vi "test_232-GNSS_gmap.vi"() -> ()   [LabVIEW 2019]
uses:
  Ctrl/gnss_config.ctl
  C:/Users/wego/Documents/GitHub/Ycar/LabVIEW/Gmap/dll/GMap.NET.WindowsForms.dll
  Gmap/dll/GMap.NET.WindowsForms.dll
  Ctrl/ublox-ui_main.ctl
  Ctrl/cmd_common.ctl
  Gmap/gmap_fgv-cmd.ctl
  Gmap/marker_info.ctl
panel:
  in  "탭":enum32{"Main", "설정"}(tab)
  in  "GMapControl":refnum<k24>(container)
  out "TM graph":T1(graph)
  in  "stop":bool
  in  "zoom":dbl(slide) scale=3.0..20.0
  in  "gmap center":bool
  in  "PinDropMrkr":T2(ring)=enum."red_dot" caption="Pin Drop Marker"
  out "error out":errorcluster
  out "n":i32
  out "read_buffer raw":string
  out "Arr-size":i32
  out "xcenter_TM":dbl
  out "ycenter_TM":dbl
  out "R_TM":dbl
  out "ublox info":T3 {"HDOP" scale=0.0..10.0; "PDOP" scale=0.0..10.0; "2D Acc.m" scale=0.0..10.0; "Latitude" format="%.9f"; "Longitude" format="%.9f"; "3D Acc.m" scale=0.0..10.0}
  in  "Map Lon":dbl format="%.11f"
  in  "Map Lat":dbl format="%.11f"
  out "read_buffer":string
  in  "GNSS cfg":T4={"Port"="COM10", "heading select"="", "PwrPak7_mode select"=[], "rate"=115200}
  out "buffer n":u32(graph)
  in  "Lon Dbclk":dbl format="%.11f"
  in  "Lat Dbclk":dbl format="%.11f"
  out "val":bool
  in  "sel":T5(ring)=enum."GxGGA"
  in  "index latlong":T6={"lat_index"=1, "lon_index"=3, "heading index"=0}
  in  "log":bool
  out "TM array":cluster{"Y(E)":dbl, "X(N)":dbl}[](array[cluster])
  in  "arr limit":i32=200
  # "GNSS/GPS Test Program"
  # "GPS/GNSS 테스트 프로그램"
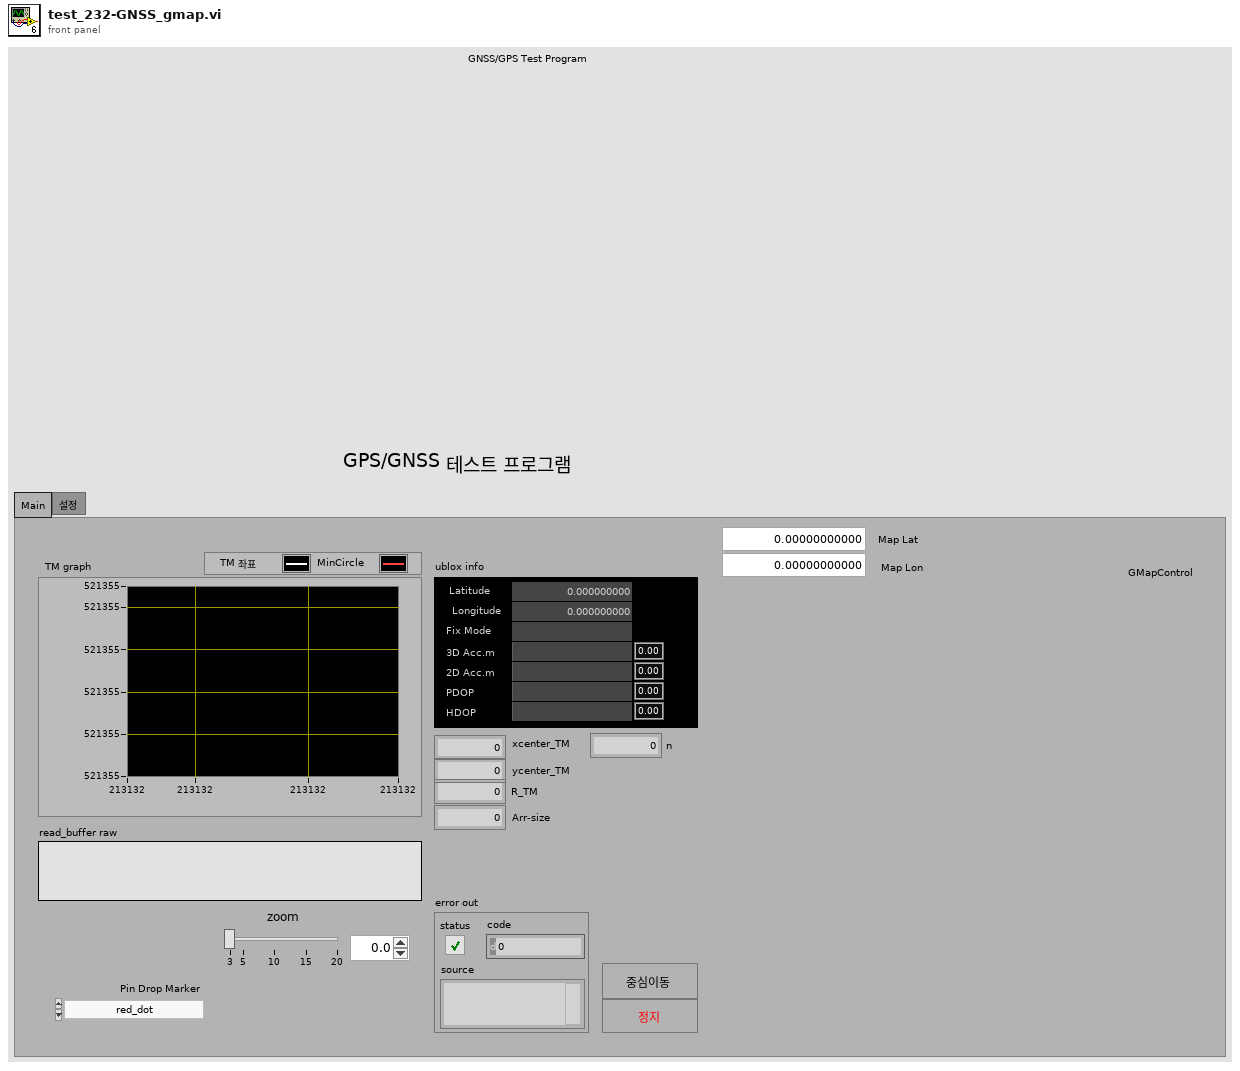
[diagram p1: front panel]
types:
  T1 = cluster{"TM array":cluster{"Y(E)":dbl, "X(N)":dbl}[]}[]
  T2 = enum16{"none", "arrow", "blue", "blue_small", "blue_dot", "blue_pushpin", "brown_small", "gray_small", "green", "green_small", "green_dot", "green_pushpin", "green_big_go", "yellow", "yellow_small", "yellow_dot", "yellow_big_pause", "yellow_pushpin", "lightblue", "lightblue_dot", "lightblue_pushpin", "orange", "orange_small", "orange_dot", "pink", "pink_dot", "pink_pushpin", "purple", "purple_small", "purple_dot", "purple_pushpin", "red", "red_small", "red_dot", "red_pushpin", "red_big_stop", "black_small", "white_small"}
  T3 = typedef "ublox-ui_main.ctl" = cluster{"Latitude":dbl, "Longitude":dbl, "Fix Mode":string, "3D Acc.m":dbl, "2D Acc.m":dbl, "PDOP":dbl, "HDOP":dbl}
  T4 = typedef "gnss_config.ctl" = cluster{"Port":refnum<visa-resource-name>, "heading select":string, "PwrPak7_mode select":string[], "rate":u32}
  T5 = enum16{"GxDTM", "GxGBS", "GxGGA", "GxGLL", "GxGNS", "GxGRS", "GxGSA", "GxGST", "GxGSV", "GxRLM", "GxRMC", "GxTHS", "GxTXT", "GxVLW", "GxVTG", "GxZDA"}
  T6 = cluster{"lat_index":i32, "lon_index":i32, "heading index":i32}
  T7 = typedef "cmd_common.ctl" = enum16{"read", "write"}
  T8 = cluster{"Map Lat":refnum<vi>, "Map Lon":refnum<vi>, "Lat Dbclk":refnum<vi>, "Lon Dbclk":refnum<vi>, "zoom":refnum<vi>, "PinDropMrkr":refnum<vi>}
  T9 = typedef "gmap_fgv-cmd.ctl" = enum16{"marker type change", "save_image", "coll of points", "zoom n center markers", "add overlay reference", "read", "zoom", "set position by keyword", "set map provider", "map provider update", "create", "add marker", "clear marker", "close"}
  T10 = typedef "marker_info.ctl" = cluster{"arrLatLngActv":dbl[], "type":i32}
  T11 = cluster{"TM array":cluster{"Y(E)":dbl, "X(N)":dbl}[]}
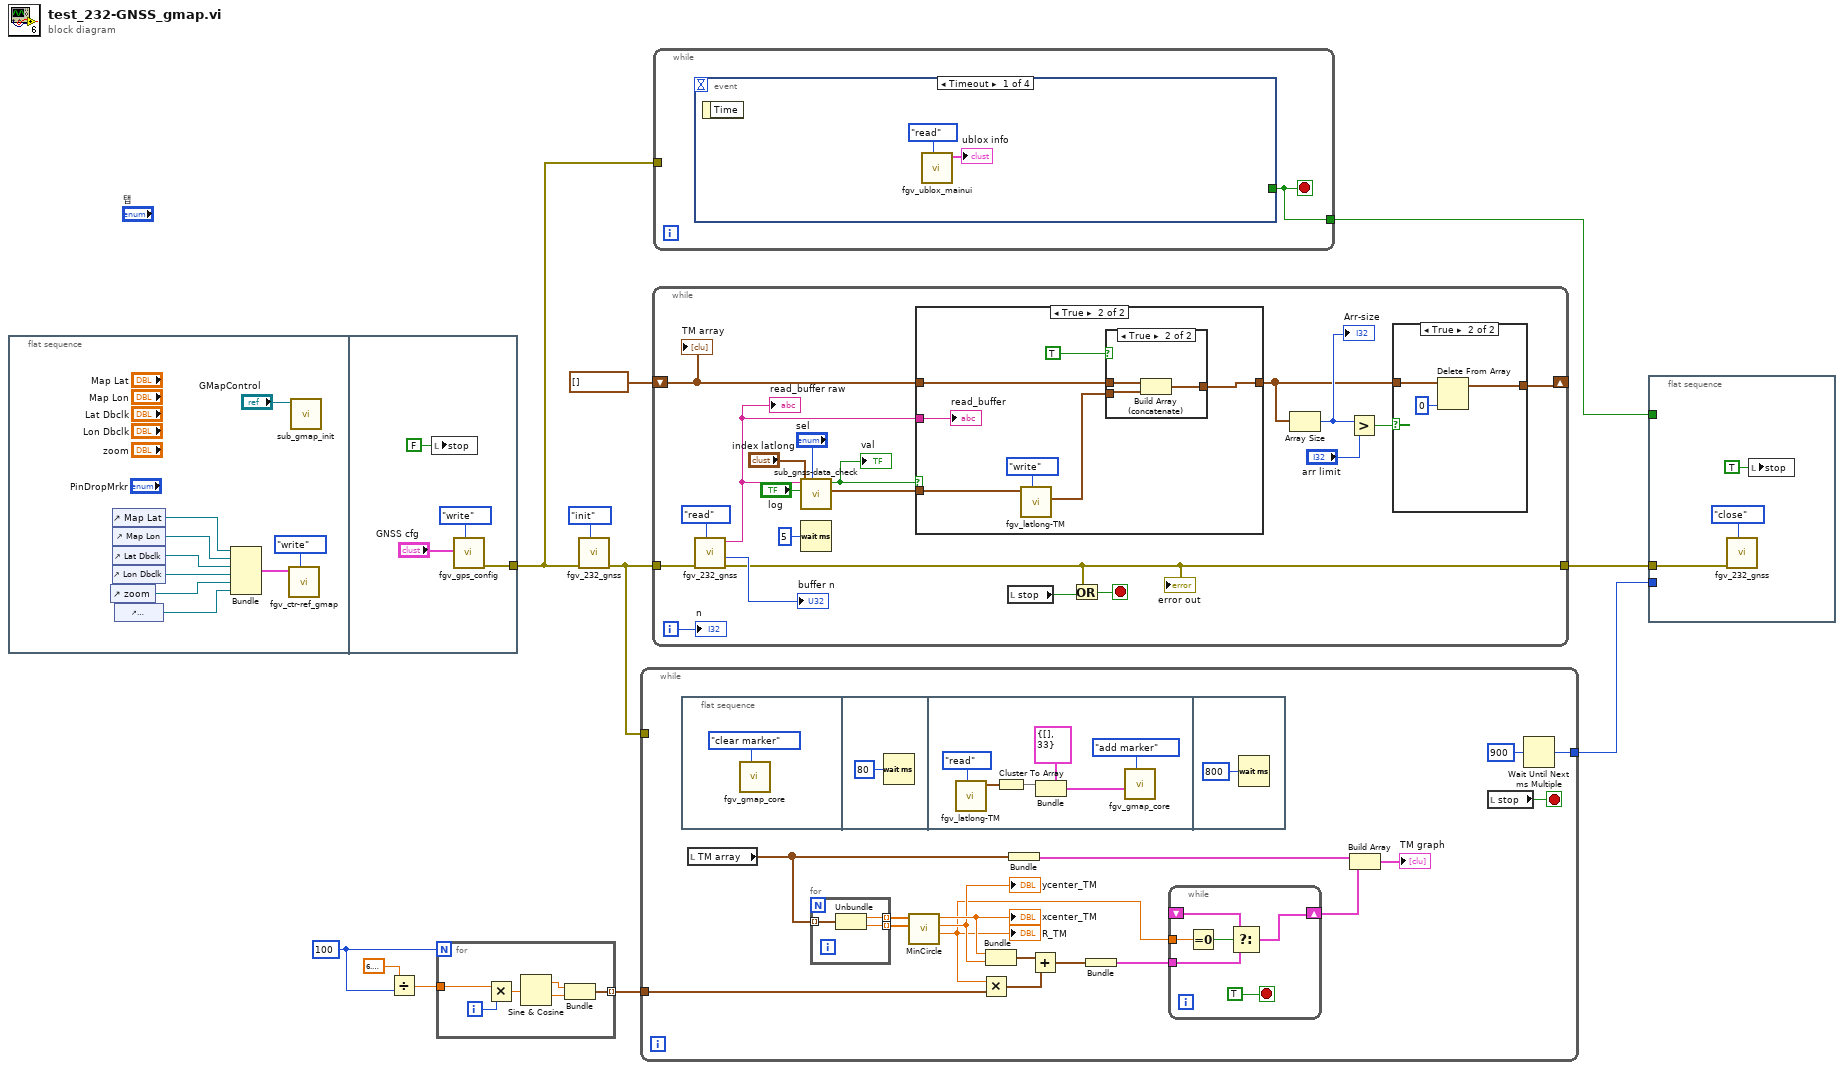
[diagram p0: block diagram]
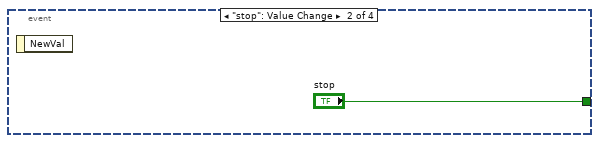
[diagram p2: hidden frame]
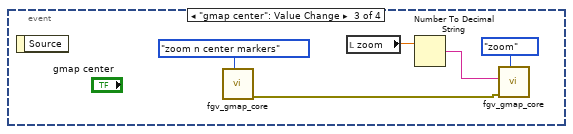
[diagram p3: hidden frame]
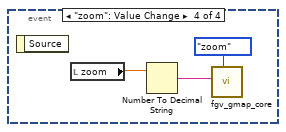
[diagram p4: hidden frame]
diagram:
  w3 = 100
  n1 = flat-sequence {
    tunnel: [w23] -> w7
    frame #0 {
      n2 = control-ref of="zoom"() -> (w13:refnum<vi>)
      n3 = control-ref of="Map Lat"() -> (w17:refnum<vi>)
      n4 = control-ref of="Map Lon"() -> (w16:refnum<vi>)
      n5 = control-ref of="Lat Dbclk"() -> (w15:refnum<vi>)
      n6 = control-ref of="Lon Dbclk"() -> (w14:refnum<vi>)
      n7 = control-ref of="PinDropMrkr"() -> (w12:refnum<vi>)
      n8 = Bundle("Map Lat"=w17, "Map Lon"=w16, "Lat Dbclk"=w15, "Lon Dbclk"=w14, "zoom"=w13, "PinDropMrkr"=w12) -> (w19:T8)  [unwired: 1 in]
      n9 = call "fgv_ctr-ref_gmap.vi"("cmd"=cmd_common."write", "ref in"=w19) -> ()  [unwired: 9 in, 1 out]
      n10 = call "sub_gmap_init.vi"("GMapControl"="GMapControl") -> ()  [unwired: 10 in, 1 out]
    }
    frame #1 {
      n11 = local write "stop"(FALSE ("정지")) -> ()
      n12 = call "fgv_gps_config.vi"("cmd"=enum16{"read", "write"}."write", "GNSS cfg"="GNSS cfg") -> ("error out"=w23:errorcluster)  [unwired: 8 in, 1 out]
    }
  }
  n13 = Divide(x=6.283185307179586, y=w3) -> (x/y=w4:dbl)
  n14 = for {
    N: w3 -> [_]
    tunnel: w4 -> [w29]
    tunnel: [w25] -> w1 mode=indexing
    i -> [w30]
    n15 = Multiply(x=w29, y=w30) -> (x*y=w28:dbl)
    n16 = Sine & Cosine(0:w28) -> (1:w27:dbl, 2:w26:dbl)
    n17 = Bundle(w27, w26) -> (w25:cluster{dbl, dbl})  [unwired: 1 in]
  }
  n18 = call "fgv_232_gnss.vi"("cmd"=enum16{"init", "read", "write", "close"}."init", "error in"=w7) -> ("error out"=w8:errorcluster)  [unwired: 7 in, 2 out]
  n19 = while {
    tunnel: w8 -> [_]
    tunnel: [w45] -> w6
    tunnel: w1 -> [w40]
    stop <- w47 stop-if-true
    n20 = flat-sequence {
      frame #0 {
        n21 = call "fgv_gmap_core.vi"("cmd"=gmap_fgv-cmd."clear marker") -> ()  [unwired: 7 in, 4 out]
      }
      frame #1 {
        n22 = Wait (ms)(milliseconds to wait=u32 80 ("대기 시간 (ms)")) -> ()  [unwired: 1 out]
      }
      frame #2 {
        n23 = call "fgv_latlong-TM.vi"("cmd"=enum16{"write", "read"}."read") -> ("latlong out"=w59:cluster{"lat":dbl, "long":dbl})  [unwired: 9 in, 1 out]
        n24 = Cluster To Array(cluster=w59) -> (array=w63:dbl[])
        n25 = Bundle(cluster=T10 {"arrLatLngActv"=[], "type"=33} ("marker_info"), "arrLatLngActv"=w63) -> (w61:T10)  [unwired: 1 in]
        n26 = call "fgv_gmap_core.vi"("cmd"=gmap_fgv-cmd."add marker", "marker_info"=w61) -> ()  [unwired: 6 in, 4 out]
      }
      frame #3 {
        n27 = Wait (ms)(milliseconds to wait=u32 800 ("대기 시간 (ms)")) -> ()  [unwired: 1 out]
      }
    }
    n28 = local read "TM array"() -> (w36:cluster{"Y(E)":dbl, "X(N)":dbl}[])
    n29 = for {
      tunnel: [w56] -> w44 mode=indexing
      tunnel: [w55] -> w43 mode=indexing
      tunnel: w36 -> [w54] mode=indexing
      n30 = Unbundle(w54) -> ("Y(E)"=w56:dbl, "X(N)"=w55:dbl)
    }
    n31 = call "MinCircle.vi"("y"=w43, "x"=w44) -> ("r"=w31:dbl, "yc"=w41:dbl, "xc"=w42:dbl)  [unwired: 6 in, 1 out]
    "xcenter_TM" <- w42
    "ycenter_TM" <- w41
    "R_TM" <- w31
    n32 = Multiply(x=w31, y=w40) -> (x*y=w39:cluster{dbl, dbl}[])
    n33 = Bundle("xc"=w42, "yc"=w41) -> (w38:cluster{"xc":dbl, "yc":dbl})  [unwired: 1 in]
    n34 = Bundle("TM array"=w36) -> (w35:T11)  [unwired: 1 in]
    n35 = Add(x=w38, y=w39) -> (x+y=w37:cluster{dbl, dbl}[])
    n36 = Bundle(w37) -> (w33:cluster{cluster{dbl, dbl}[]})  [unwired: 1 in]
    n37 = while {
      shift-right: [w48] -> w32
      shift-left: _ -> [w50]
      tunnel: w31 -> [w52]
      tunnel: w33 -> [w49]
      stop <- TRUE stop-if-true
      n38 = Equal To 0?(x=w52) -> (x = 0?=w51:bool)
      n39 = Select(t=w50, s=w51, f=w49) -> (s? t:f=w48:cluster{cluster{dbl, dbl}[]})
    }
    n40 = Build Array(w35, w32) -> (→"TM graph":T1)
    n41 = local read "stop"() -> (w47:bool)
    n42 = Wait Until Next ms Multiple(millisecond multiple=u32 900 ("ms 배수")) -> (millisecond timer value=w45:u32)
  }
  n43 = while {
    shift-right: [w66] -> _
    shift-left: cluster{"Y(E)":dbl, "X(N)":dbl}[] [] -> [w82]
    tunnel: w8 -> [w83]
    tunnel: [w76] -> w10
    i -> [w78]
    stop <- w75 stop-if-true
    n44 = call "fgv_232_gnss.vi"("cmd"=enum16{"init", "read", "write", "close"}."read", "error in"=w83) -> ("error out"=w76:errorcluster, "byte n"=→"buffer n":u32, "read_buffer"=w80:string)  [unwired: 7 in]
    "error out" <- w76
    "read_buffer raw" <- w80
    n45 = call "sub_gnss-data_check.vi"("sel"="sel", "index cluster"="index latlong", "log"="log", "gnss str"=w80) -> ("LatLong"=w74:cluster{dbl, dbl}, "val"=w73:bool)  [unwired: 5 in, 1 out]
    "val" <- w73
    n46 = Wait (ms)(milliseconds to wait=u32 5 ("대기 시간 (ms)")) -> ()  [unwired: 1 out]
    n47 = case shown="True" w73 {
      tunnel: [w90 w97] -> w67
      tunnel: w82 -> [w90 w96]
      tunnel: w80 -> [_ w95]
      tunnel: w74 -> [_ w92]
      frame False {
      }
      frame True {
        n48 = call "fgv_latlong-TM.vi"("cmd"=enum16{"write", "read"}."write", "latlong"=w92) -> ("tm out"=w91:cluster{"YE":dbl, "XN":dbl})  [unwired: 8 in, 1 out]
        n49 = case shown="True" TRUE {
          tunnel: [w98 w101] -> w97
          tunnel: w96 -> [w98 w100]
          tunnel: w91 -> [_ w99]
          frame False {
          }
          frame True {
            n50 = Build Array (concatenate)(w100, w99) -> (w101:cluster{"YE":dbl, "XN":dbl}[])
          }
        }
        "read_buffer" <- w95
      }
    }
    n51 = local read "stop"() -> (w77:bool)
    n52 = Or(x=w76, y=w77) -> (x .or. y?=w75:bool)
    n53 = Array Size(array=w67) -> (size(s)=w70:i32)
    "Arr-size" <- w70
    n54 = Greater?(x=w70, y="arr limit") -> (0:w68:bool)
    n55 = case shown="True" w68 {
      tunnel: w67 -> [w86 w88]
      tunnel: [w86 w87] -> w66
      frame False {
      }
      frame True {
        n56 = Delete From Array(array=w88, index=0) -> (array with subset deleted=w87:cluster{"YE":dbl, "XN":dbl}[])  [unwired: 1 in, 1 out]
      }
    }
    "n" <- w78
    "TM array" <- w82
  }
  n57 = while {
    tunnel: w7 -> [_]
    tunnel: [w102] -> w5
    stop <- w102 stop-if-true
    n58 = event shown="[0] Timeout" {
      selector: _ -> [_ _ _ _]
      dyn-events: _ -> [_ _ _ _]
      timeout: _ -> [_ _ _ _]
      tunnel: [_ "stop" _ _] -> w102
      event Timeout {
        n59 = event-data() -> ()  [unwired: 1 in, 1 out]
        n60 = call "fgv_ublox_mainui.vi"("cmd"=cmd_common."read") -> ("MainUI ublox out"=→"ublox info":T3)  [unwired: 10 in]
      }
      event "stop": Value Change {
        n61 = event-data() -> ()  [unwired: 1 in, 1 out]
      }
      event "gmap center": Value Change {
        n62 = event-data() -> ()  [unwired: 1 in, 1 out]
        n63 = call "fgv_gmap_core.vi"("cmd"=gmap_fgv-cmd."zoom n center markers") -> ("error out"=w106:errorcluster)  [unwired: 7 in, 3 out]
        n64 = local read "zoom"() -> (w109:dbl)
        n65 = Number To Decimal String(number=w109) -> (decimal integer string=w108:string)  [unwired: 1 in]
        n66 = call "fgv_gmap_core.vi"(7:"cmd"=gmap_fgv-cmd."zoom" ("cmd"), "error in"=w106, 10:"cmd"=w108) -> ()  [unwired: 5 in, 4 out]
      }
      event "zoom": Value Change {
        n67 = event-data() -> ()  [unwired: 1 in, 1 out]
        n68 = local read "zoom"() -> (w112:dbl)
        n69 = Number To Decimal String(number=w112) -> (decimal integer string=w111:string)  [unwired: 1 in]
        n70 = call "fgv_gmap_core.vi"(7:"cmd"=gmap_fgv-cmd."zoom" ("cmd"), 10:"cmd"=w111) -> ()  [unwired: 6 in, 4 out]
      }
    }
  }
  n71 = flat-sequence {
    tunnel: w10 -> [w115]
    tunnel: w6 -> [_]
    tunnel: w5 -> [_]
    frame #0 {
      n72 = call "fgv_232_gnss.vi"("cmd"=enum16{"init", "read", "write", "close"}."close", "error in"=w115) -> ()  [unwired: 7 in, 3 out]
      n73 = local write "stop"(TRUE ("stop")) -> ()
    }
  }
